vi "Flip.vi"(8 "error in":errorcluster, 11 "Screen Pointer":u32 format="%.0x") -> (0 "error out":errorcluster, 3 "Return":i32)   [LabVIEW 2015]
uses:
  DLL/SDL2.dll
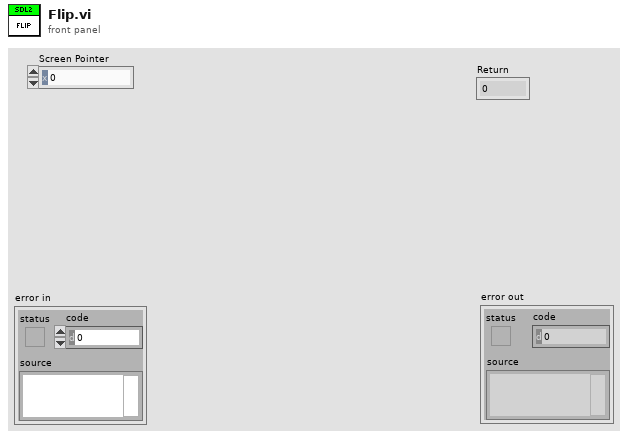
[diagram p1: front panel]
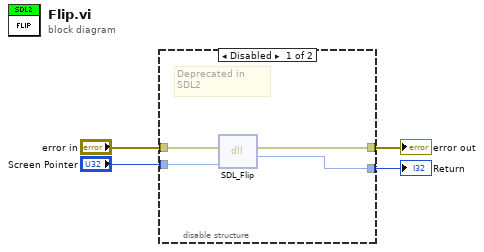
[diagram p0: block diagram]
diagram:
  n1 = disable-structure shown="Disabled" {
    disable-tunnel: "error in" -> [w8 _]
    disable-tunnel: [w7 _] -> w3
    disable-tunnel: "Screen Pointer" -> [w6 _]
    disable-tunnel: [w5 _] -> w1
    frame Disabled {
      # "Deprecated in SDL2"
      n2 = dll-call lib="C:/dev/PGS/LabSDL2/Source/Libraries/LibSDL2 Wrapper/DLL/SDL2.dll" fn="SDL_Flip"(error in=w8, "screen"=w6) -> (error out=w7:errorcluster, "return type"=w5:i32)  [unwired: 3 in, 1 out]
    }
    frame Enabled {
    }
  }
  "error out" <- w3
  "Return" <- w1
